vi "Compute Order and Cutoffs.vi"(6 "fs [Hz]":dbl=1.0 format="%.2f", 7 "filter type":T5, 8 "error in (no error)":errorcluster, 9 "design method":T4(ring)=enum."Elliptic", 10 "ripple specs":T2={"passband"=0.1, "stopband"=40.0, "dB/linear? (T: dB)"=TRUE}, 11 "freq specs [Hz]":T3) -> (0 "error out":errorcluster, 1 "low cutoff freq: fl":dbl, 2 "high cutoff freq: fh":dbl, 3 "n":i32=5, 4 "ripples [dB]":T1 {"stopband atten" format="%.2f"; "passband ripple" format="%.2f"})   [LabVIEW 2020, in "NI_AAL_Filter.lvlib"]
uses:
  <vilib>/Analysis/NI_AAL_Filter.lvlib
  <vilib>/Analysis/3filter.llb/Filter Passband Type.ctl
  <vilib>/Analysis/3filter.llb/Filter Frequence Specification (Design).ctl
  <vilib>/Analysis/3filter.llb/Filter Ripple Specification (Design).ctl
  <vilib>/Analysis/NI_AALBase.lvlib
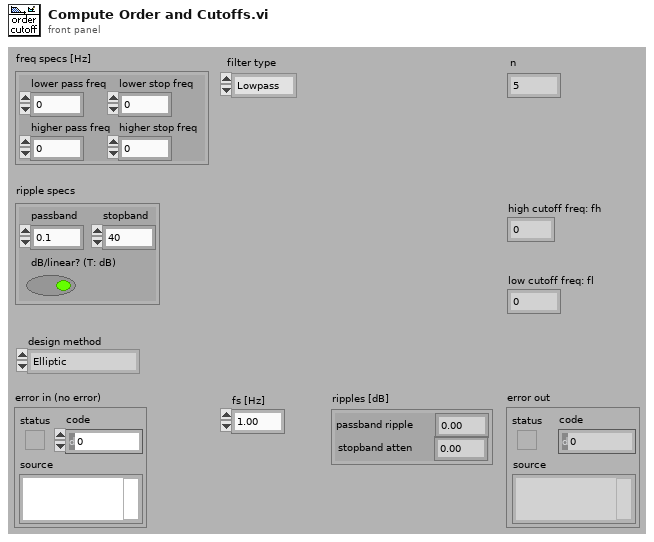
[diagram p1: front panel]
types:
  T1 = cluster{"passband ripple":dbl, "stopband atten":dbl}
  T2 = typedef "NI_AAL_Filter.lvlib/Filter Ripple Specification (Design).ctl" = cluster{"passband":dbl, "stopband":dbl, "dB/linear? (T: dB)":bool}
  T3 = typedef "NI_AAL_Filter.lvlib/Filter Frequence Specification (Design).ctl" = cluster{"lower pass freq":dbl, "lower stop freq":dbl, "higher pass freq":dbl, "higher stop freq":dbl}
  T4 = enum16{"Butterworth", "Chebyshev", "Inverse Chebyshev", "Elliptic", "Bessel"}
  T5 = typedef "NI_AALBase.lvlib/Filter Passband Type.ctl" = enum32{"Lowpass", "Highpass", "Bandpass", "Bandstop"}
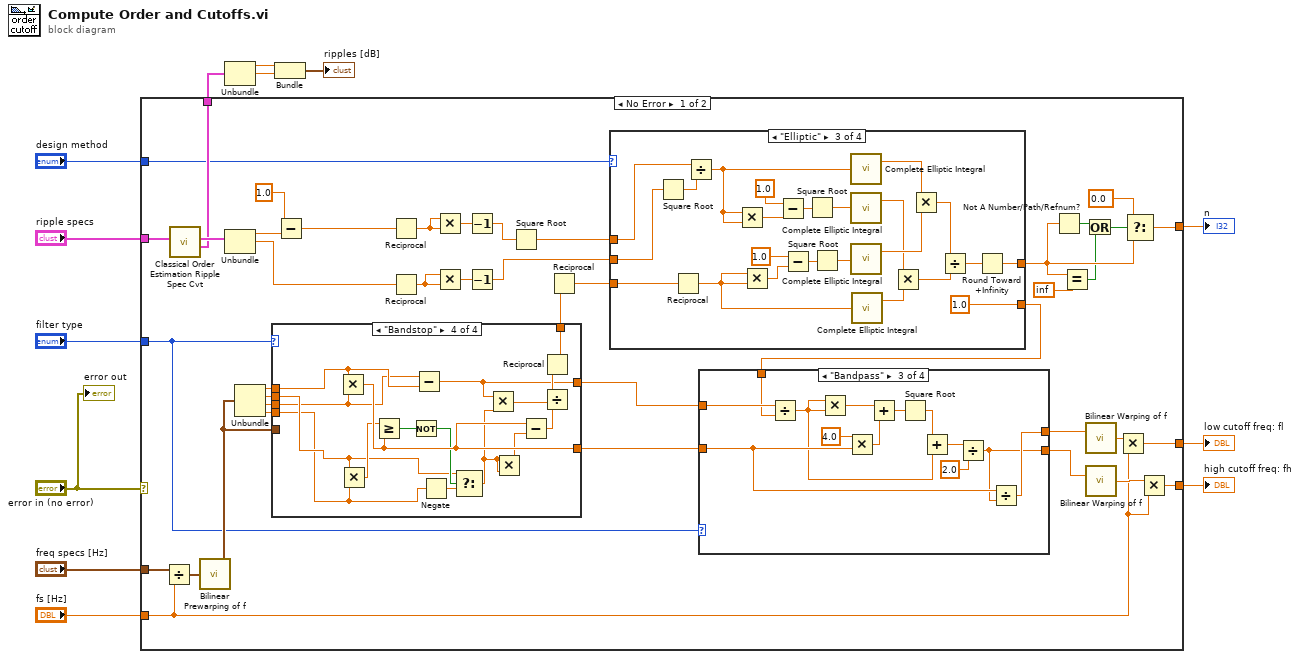
[diagram p0: block diagram]
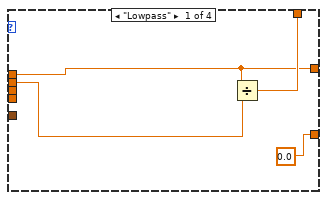
[diagram p2: hidden frame]
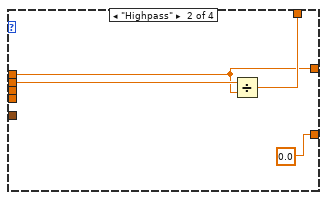
[diagram p3: hidden frame]
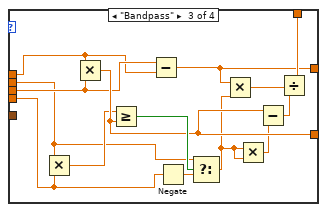
[diagram p4: hidden frame]
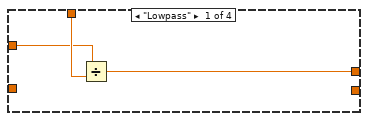
[diagram p5: hidden frame]
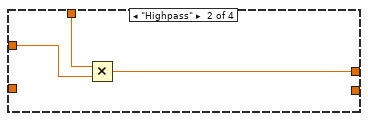
[diagram p6: hidden frame]
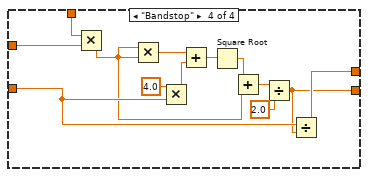
[diagram p7: hidden frame]
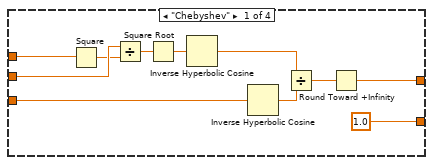
[diagram p8: hidden frame]
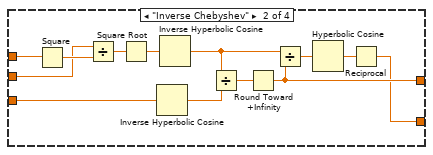
[diagram p9: hidden frame]
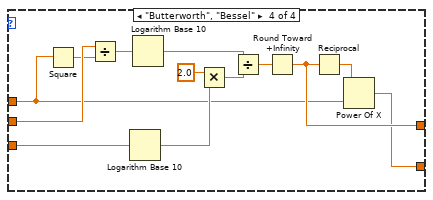
[diagram p10: hidden frame]
diagram:
  n1 = case shown="No Error" "error in (no error)" {
    tunnel: "filter type" -> [w23 _]
    tunnel: [w14 _] -> w12
    tunnel: "freq specs [Hz]" -> [w37 _]
    tunnel: "fs [Hz]" -> [w17 _]
    tunnel: "ripple specs" -> [w35 _]
    tunnel: [w22 _] -> w5
    tunnel: [w20 _] -> w7
    tunnel: [w16 _] -> w6
    tunnel: "design method" -> [w15 _]
    frame No Error {
      n2 = Divide(x=w37, y=w17) -> (x/y=w31:T3)
      n3 = call <vilib>:"Classical Order Estimation Ripple Spec Cvt.vi"("ripple specs"=w35) -> ("ripple specs (dB)"=w22:T2, "ripple specs (linear)"=w34:T2)  [unwired: 9 out]
      n4 = call <vilib>:"Bilinear Prewarping of f.vi"("freq specs [Hz]"=w31) -> ("prewarped freq specs [Hz]"=w30:T3)
      n5 = Unbundle(w34) -> ("passband"=w33:dbl, "stopband"=w24:dbl)  [unwired: 1 out]
      n6 = Unbundle(w30) -> ("lower pass freq"=w29:dbl, "lower stop freq"=w28:dbl, "higher pass freq"=w27:dbl, "higher stop freq"=w26:dbl)
      n7 = case shown="\"Bandstop\"" w23 {
        tunnel: [w59 w63 w76 w82] -> w51
        tunnel: [w57 w60 w75 w91] -> w50
        tunnel: [0.0 0.0 w74 w90] -> w49
        tunnel: w30 -> [_ _ _ _]
        tunnel: w29 -> [w57 w60 w65 w81]
        tunnel: w28 -> [w56 w61 w66 w80]
        tunnel: w27 -> [_ _ w68 w79]
        tunnel: w26 -> [_ _ w67 w78]
        frame "Lowpass" {
          n8 = Divide(x=w57, y=w56) -> (x/y=w59:dbl)
        }
        frame "Highpass" {
          n9 = Divide(x=w61, y=w60) -> (x/y=w63:dbl)
        }
        frame "Bandpass" {
          n10 = Multiply(x=w66, y=w67) -> (x*y=w73:dbl)
          n11 = Multiply(x=w65, y=w68) -> (x*y=w74:dbl)
          n12 = Greater Or Equal?(x=w73, y=w74) -> (x >= y?=w77:bool)
          n13 = Subtract(x=w68, y=w65) -> (x-y=w75:dbl)
          n14 = Negate(x=w67) -> (-x=w72:dbl)
          n15 = Select(t=w66, s=w77, f=w72) -> (s? t:f=w71:dbl)
          n16 = Multiply(x=w75, y=w71) -> (x*y=w69:dbl)
          n17 = Multiply(x=w71, y=w71) -> (x*y=w64:dbl)
          n18 = Subtract(x=w74, y=w64) -> (x-y=w70:dbl)
          n19 = Divide(x=w69, y=w70) -> (x/y=w76:dbl)
        }
        frame "Bandstop" {
          n20 = Multiply(x=w81, y=w79) -> (x*y=w90:dbl)
          n21 = Multiply(x=w80, y=w78) -> (x*y=w89:dbl)
          n22 = Greater Or Equal?(x=w89, y=w90) -> (x >= y?=w93:bool)
          n23 = Not(x=w93) -> (.not. x?=w83:bool)
          n24 = Subtract(x=w79, y=w81) -> (x-y=w91:dbl)
          n25 = Negate(x=w78) -> (-x=w88:dbl)
          n26 = Select(t=w80, s=w83, f=w88) -> (s? t:f=w87:dbl)
          n27 = Multiply(x=w91, y=w87) -> (x*y=w84:dbl)
          n28 = Multiply(x=w87, y=w87) -> (x*y=w86:dbl)
          n29 = Subtract(x=w90, y=w86) -> (x-y=w85:dbl)
          n30 = Divide(x=w84, y=w85) -> (x/y=w92:dbl)
          n31 = Reciprocal(x=w92) -> (1/x=w82:dbl)
        }
      }
      n32 = Subtract(x=1.0, y=w33) -> (x-y=w25:dbl)
      n33 = Reciprocal(x=w25) -> (1/x=w44:dbl)
      n34 = Reciprocal(x=w24) -> (1/x=w54:dbl)
      n35 = Multiply(x=w44, y=w44) -> (x*y=w45:dbl)
      n36 = Multiply(x=w54, y=w54) -> (x*y=w53:dbl)
      n37 = Decrement(x=w45) -> (x-1=w46:dbl)
      n38 = Decrement(x=w53) -> (x-1=w55:dbl)
      n39 = Square Root(x=w46) -> (sqrt(x)=w47:dbl)
      n40 = Reciprocal(x=w51) -> (1/x=w52:dbl)
      n41 = case shown="\"Elliptic\"" w15 {
        tunnel: w52 -> [w130 w142 w151 w182]
        tunnel: [1.0 w137 1.0 w173] -> w48
        tunnel: w47 -> [w135 w144 w154 w175]
        tunnel: [w126 w140 w153 w176] -> w41
        tunnel: w55 -> [w134 w143 w150 w185]
        frame "Chebyshev" {
          n42 = Square(x=w135) -> (x^2=w133:dbl)
          n43 = Divide(x=w134, y=w133) -> (x/y=w132:dbl)
          n44 = Square Root(x=w132) -> (sqrt(x)=w131:dbl)
          n45 = Inverse Hyperbolic Cosine(1:w131) -> (0:w129:dbl)
          n46 = Inverse Hyperbolic Cosine(1:w130) -> (0:w128:dbl)
          n47 = Divide(x=w129, y=w128) -> (x/y=w127:dbl)
          n48 = Round Toward +Infinity(x=w127) -> (ceil(x): smallest int >= x=w126:dbl)
        }
        frame "Inverse Chebyshev" {
          n49 = Square(x=w144) -> (x^2=w149:dbl)
          n50 = Divide(x=w143, y=w149) -> (x/y=w148:dbl)
          n51 = Square Root(x=w148) -> (sqrt(x)=w147:dbl)
          n52 = Inverse Hyperbolic Cosine(1:w142) -> (0:w146:dbl)
          n53 = Inverse Hyperbolic Cosine(1:w147) -> (0:w141:dbl)
          n54 = Divide(x=w141, y=w146) -> (x/y=w145:dbl)
          n55 = Round Toward +Infinity(x=w145) -> (ceil(x): smallest int >= x=w140:dbl)
          n56 = Divide(x=w141, y=w140) -> (x/y=w139:dbl)
          n57 = Hyperbolic Cosine(1:w139) -> (0:w138:dbl)
          n58 = Reciprocal(x=w138) -> (1/x=w137:dbl)
        }
        frame "Elliptic" {
          n59 = Square Root(x=w150) -> (sqrt(x)=w172:dbl)
          n60 = Reciprocal(x=w151) -> (1/x=w155:dbl)
          n61 = Divide(x=w154, y=w172) -> (x/y=w164:dbl)
          n62 = Multiply(x=w164, y=w164) -> (x*y=w166:dbl)
          n63 = Multiply(x=w155, y=w155) -> (x*y=w170:dbl)
          n64 = Subtract(x=1.0, y=w166) -> (x-y=w167:dbl)
          n65 = Subtract(x=1.0, y=w170) -> (x-y=w169:dbl)
          n66 = Square Root(x=w167) -> (sqrt(x)=w163:dbl)
          n67 = Square Root(x=w169) -> (sqrt(x)=w168:dbl)
          n68 = call <vilib>:"Complete Elliptic Integral.vi"("k'"=w164) -> ("cei(k)"=w162:dbl)  [unwired: 1 out]
          n69 = call <vilib>:"Complete Elliptic Integral.vi"("k'"=w163) -> ("cei(k)"=w156:dbl)  [unwired: 1 out]
          n70 = call <vilib>:"Complete Elliptic Integral.vi"("k'"=w168) -> ("cei(k)"=w161:dbl)  [unwired: 1 out]
          n71 = call <vilib>:"Complete Elliptic Integral.vi"("k'"=w155) -> ("cei(k)"=w160:dbl)  [unwired: 1 out]
          n72 = Multiply(x=w156, y=w160) -> (x*y=w159:dbl)
          n73 = Multiply(x=w162, y=w161) -> (x*y=w158:dbl)
          n74 = Divide(x=w158, y=w159) -> (x/y=w157:dbl)
          n75 = Round Toward +Infinity(x=w157) -> (ceil(x): smallest int >= x=w153:dbl)
        }
        frame "Butterworth", "Bessel" {
          n76 = Square(x=w175) -> (x^2=w184:dbl)
          n77 = Divide(x=w185, y=w184) -> (x/y=w183:dbl)
          n78 = Logarithm Base 10(1:w182) -> (0:w181:dbl)
          n79 = Logarithm Base 10(1:w183) -> (0:w179:dbl)
          n80 = Multiply(x=2.0, y=w181) -> (x*y=w178:dbl)
          n81 = Divide(x=w179, y=w178) -> (x/y=w177:dbl)
          n82 = Round Toward +Infinity(x=w177) -> (ceil(x): smallest int >= x=w176:dbl)
          n83 = Reciprocal(x=w176) -> (1/x=w174:dbl)
          n84 = Power Of X(1:w175, 2:w174) -> (0:w173:dbl)
        }
      }
      n85 = case shown="\"Bandpass\"" w23 {
        tunnel: w50 -> [w95 w98 w112 w116]
        tunnel: w49 -> [_ _ w111 w125]
        tunnel: w48 -> [w96 w99 w104 w115]
        tunnel: [w94 w97 w101 w114] -> w21
        tunnel: [_ _ w100 w113] -> w18
        frame "Lowpass" {
          n86 = Divide(x=w95, y=w96) -> (x/y=w94:dbl)
        }
        frame "Highpass" {
          n87 = Multiply(x=w99, y=w98) -> (x*y=w97:dbl)
        }
        frame "Bandpass" {
          n88 = Divide(x=w112, y=w104) -> (x/y=w102:dbl)
          n89 = Multiply(x=w102, y=w102) -> (x*y=w103:dbl)
          n90 = Multiply(x=4.0, y=w111) -> (x*y=w106:dbl)
          n91 = Add(x=w103, y=w106) -> (x+y=w107:dbl)
          n92 = Square Root(x=w107) -> (sqrt(x)=w108:dbl)
          n93 = Add(x=w108, y=w102) -> (x+y=w109:dbl)
          n94 = Divide(x=w109, y=2.0) -> (x/y=w100:dbl)
          n95 = Divide(x=w111, y=w100) -> (x/y=w101:dbl)
        }
        frame "Bandstop" {
          n96 = Multiply(x=w115, y=w116) -> (x*y=w117:dbl)
          n97 = Multiply(x=w117, y=w117) -> (x*y=w118:dbl)
          n98 = Multiply(x=4.0, y=w125) -> (x*y=w120:dbl)
          n99 = Add(x=w118, y=w120) -> (x+y=w121:dbl)
          n100 = Square Root(x=w121) -> (sqrt(x)=w122:dbl)
          n101 = Add(x=w122, y=w117) -> (x+y=w123:dbl)
          n102 = Divide(x=w123, y=2.0) -> (x/y=w113:dbl)
          n103 = Divide(x=w125, y=w113) -> (x/y=w114:dbl)
        }
      }
      n104 = Not A Number/Path/Refnum?(number/path/refnum=w41) -> (NaN/Path/Refnum?=w43:bool)
      n105 = Equal?(x=w41, y=inf) -> (x = y?=w38:bool)
      n106 = Or(x=w43, y=w38) -> (x .or. y?=w39:bool)
      n107 = call <vilib>:"Bilinear Warping of f.vi"("f"=w21) -> ("prewarped f"=w36:dbl)
      n108 = call <vilib>:"Bilinear Warping of f.vi"("f"=w18) -> ("prewarped f"=w19:dbl)
      n109 = Multiply(x=w36, y=w17) -> (x*y=w20:dbl)
      n110 = Select(t=0.0, s=w39, f=w41) -> (s? t:f=w14:dbl)
      n111 = Multiply(x=w19, y=w17) -> (x*y=w16:dbl)
    }
    frame Error {
    }
  }
  "n" <- w12
  "low cutoff freq: fl" <- w7
  "high cutoff freq: fh" <- w6
  n112 = Unbundle(w5) -> ("passband"=w4:dbl, "stopband"=w3:dbl)  [unwired: 1 out]
  n113 = Bundle("passband"=w4, "stopband"=w3) -> (→"ripples [dB]":cluster{"passband":dbl, "stopband":dbl})  [unwired: 1 out]
  "error out" <- "error in (no error)"
